vi "Replace Multiple Wheels in Steering Frame by Name.vi"(5 "x positions":dbl[](array[numeric]), 6 "frame angles (rad)":dbl[](array[numeric]), 7 "y positions":dbl[](array[numeric]), 8 "error in (no error)":errorcluster, 9 "wheels":refnum<class "NI_Robotics_Wheel.lvclass">[](array[class]), 10 "wheel names":string[](array[string]), 11 "steering frame in":refnum<class "NI_Robotics_Steering Frame.lvclass">) -> (0 "error out":errorcluster, 1 "found?":bool[](array[boolean]), 3 "steering frame out":refnum<class "NI_Robotics_Steering Frame.lvclass">)   [LabVIEW 2017, in "NI_Robotics_Steering Frame.lvclass"]
doc: "Replaces wheels in <B>steering frame in</B> with the wheels you specify. You must manually select the polymorphic instance to use."
uses:
  <vilib>/robotics/Steering/Steering Frame/NI_Robotics_Steering Frame.lvclass
  <vilib>/robotics/Steering/Wheel/NI_Robotics_Wheel.lvclass
  <vilib>/robotics/Steering/Steering Frame/NI_Robotics_Steering Frame.lvclass/NI_Robotics_Steering Frame.ctl
  <vilib>/robotics/Steering/Wheel/NI_Robotics_Wheel.lvclass/NI_Robotics_Wheel.ctl
  <vilib>/robotics/Steering/Wheel/Get Wheel Name.vi
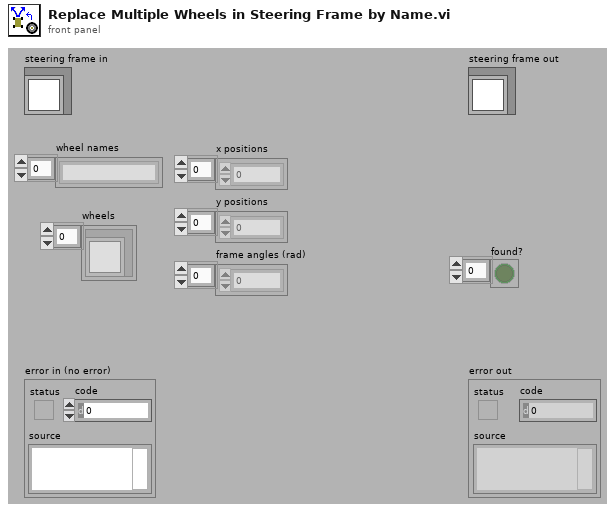
[diagram p1: front panel]
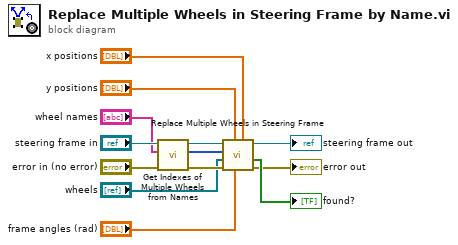
[diagram p0: block diagram]
diagram:
  n1 = call <vilib>:"Get Indexes of Multiple Wheels from Names.vi"("error in (no error)"="error in (no error)", "wheel names"="wheel names", "steering frame in"="steering frame in") -> ("error out"=w9:errorcluster, "indexes"=w10:i32[], "steering frame out"=w11:refnum<class "NI_Robotics_Steering Frame.lvclass">)  [unwired: 5 in, 1 out]
  n2 = call <vilib>:"Replace Multiple Wheels in Steering Frame.vi"("x positions"="x positions", "frame angles (rad)"="frame angles (rad)", "y positions"="y positions", "error in (no error)"=w9, "wheels"="wheels", "wheel indexes"=w10, "steering frame in"=w11) -> ("error out"=→"error out":errorcluster, "found?"=→"found?":bool[], "steering frame out"=→"steering frame out":refnum<class "NI_Robotics_Steering Frame.lvclass">)  [unwired: 2 in]
